vi "Global Send To ANN.vi"() -> ()   [LabVIEW 2020]
panel:
  in  "Send to ANN":bool
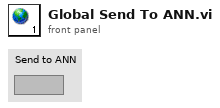
[diagram p1: front panel]
diagram:
